vi "Write Parameters to Word.vi"(8 "error in":errorcluster, 9 "parameters definitions":T1[](array[typedef]), 10 "parameters values":dbl[](array[numeric]), 11 "32-bit Word in":refnum<class "32-bit Word.lvclass">) -> (0 "error out":errorcluster, 3 "32-bit Word out":refnum<class "32-bit Word.lvclass">)   [LabVIEW 2020, in "32-bit Word.lvclass"]
uses:
  32-bit Word.lvclass
  Parameter Definition.ctl
  Encoding and Decoding/Encoding.ctl
  ARINC 429.lvclass
  Encoding and Decoding/Encoding and Decoding.lvlib
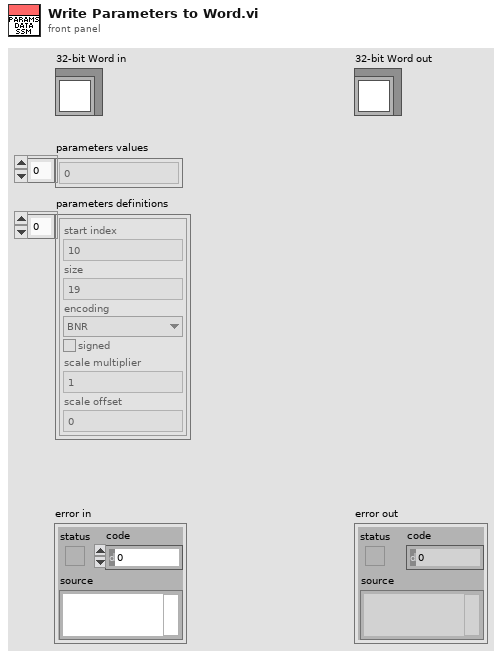
[diagram p1: front panel]
types:
  T1 = typedef "ARINC 429.lvclass/Parameter Definition.ctl" = cluster{"start index":i32, "size":i32, "encoding":T2, "signed":bool, "scale multiplier":dbl, "scale offset":dbl}
  T2 = typedef "Encoding and Decoding.lvlib/Encoding.ctl" = enum16{"BNR", "BCD", "Discrete"}
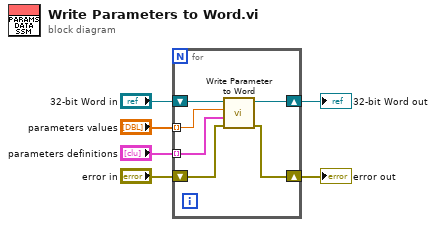
[diagram p0: block diagram]
diagram:
  n1 = for {
    shift-right: [w11] -> w5
    shift-left: "32-bit Word in" -> [w12]
    tunnel: "parameters values" -> [w10] mode=indexing
    tunnel: "parameters definitions" -> [w9] mode=indexing
    shift-right: [w7] -> w1
    shift-left: "error in" -> [w8]
    n2 = call-dynamic "Write Parameter to Word.vi"("error in"=w8, "parameter definition"=w9, "data"=w10, "32-bit Word in"=w12) -> ("error out"=w7:errorcluster, "32-bit Word out"=w11:refnum<class "32-bit Word.lvclass">)  [unwired: 6 in]
  }
  "error out" <- w1
  "32-bit Word out" <- w5
